vi "Distillation Column #2.vi"() -> ()   [LabVIEW 2017]
uses:
  Halt BioReact.vi
panel:
  in  "Cooling Water Setpoint":dbl caption="L/hr"
  in  "Main Power":bool
  out "Feed Scale":dbl caption="kg" format="%.4f"
  out "Cooling Water Flowrate":dbl caption="L/hr" format="%.1f"
  out "Reboiler Pressure":dbl caption="\"WC" format="%.1f"
  in  "stop":bool
  out "Data Point Count":i32
  in  "Specify Time between Data Points (sec)":dbl=1.0
  in  "Cancel Data Collection":bool
  in  "Specify number of data points":i16=1
  in  "Enable 3":bool
  out "Saving Data 3":bool
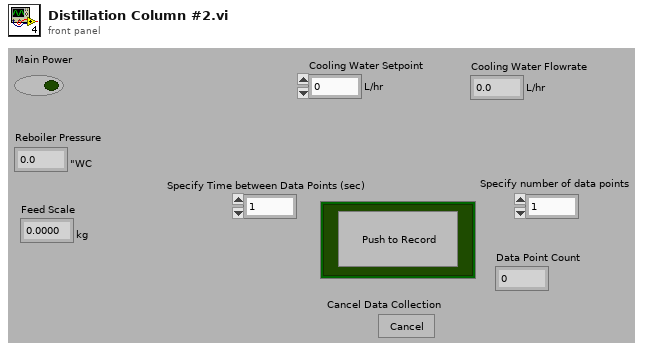
[diagram p1: front panel]
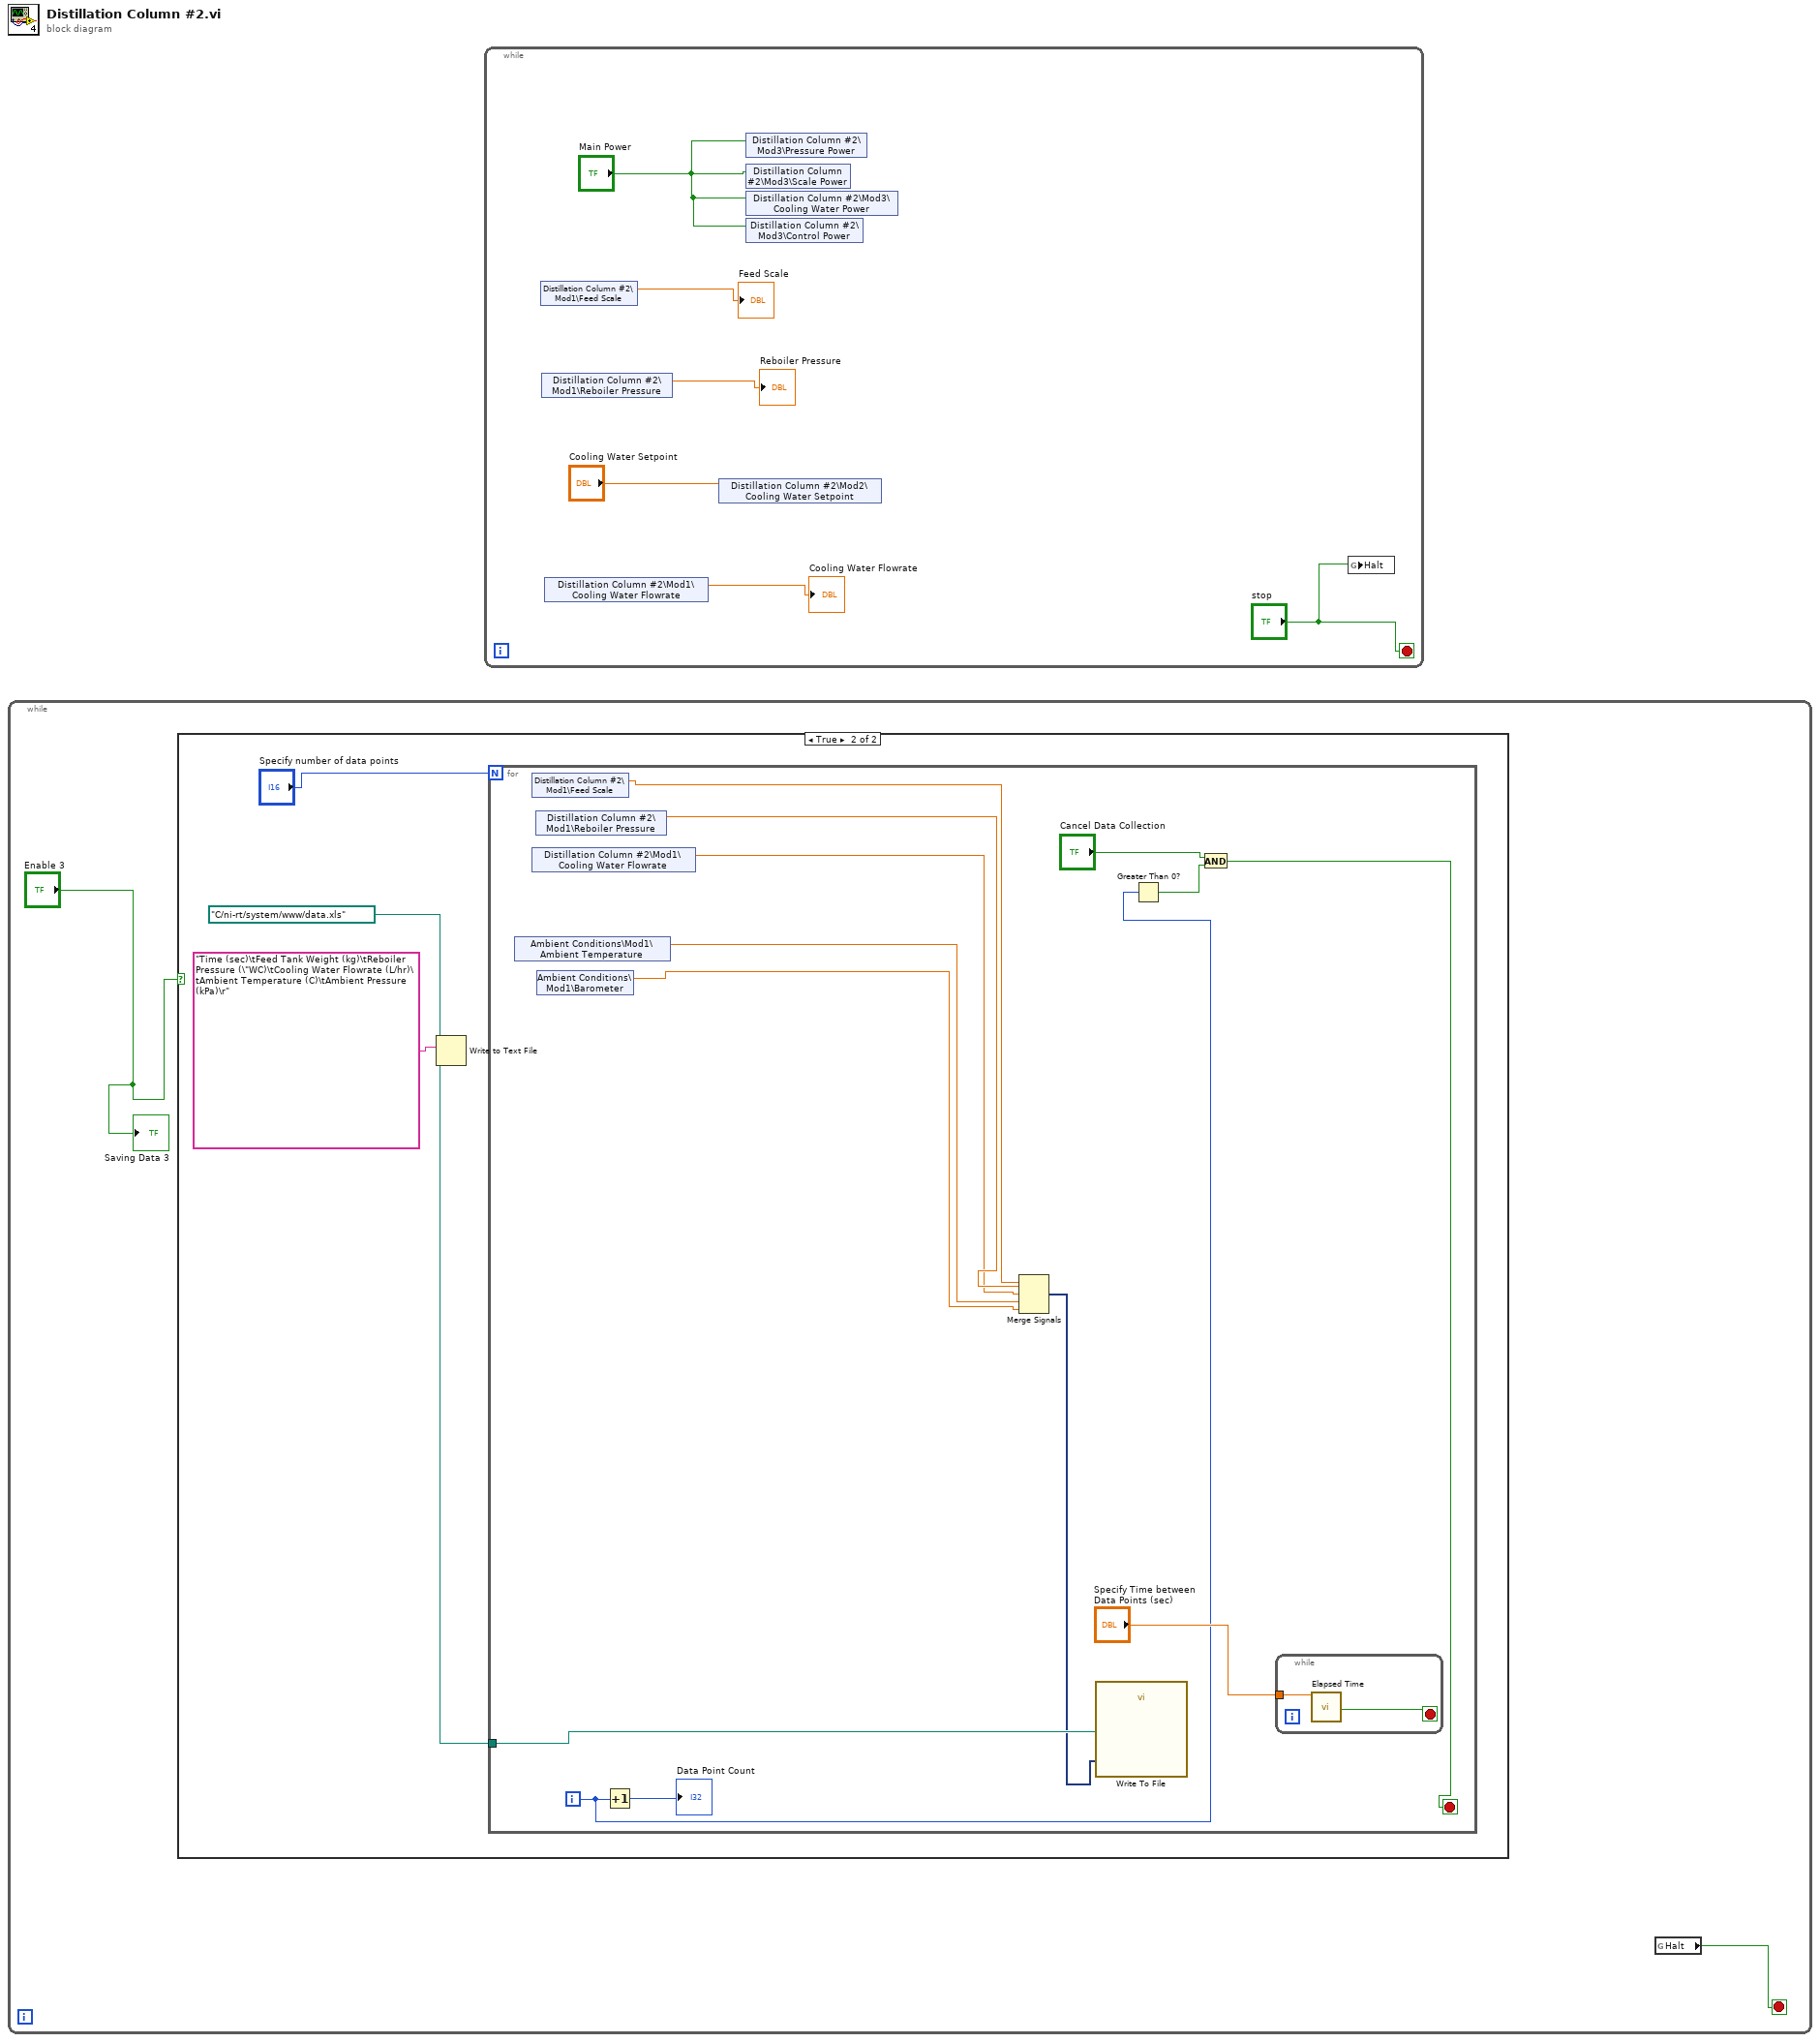
[diagram p0: block diagram]
diagram:
  n1 = while {
    stop <- w1 stop-if-true
    n2 = case shown="True" "Enable 3" {
      frame False {
      }
      frame True {
        w4 = path "C:/ni-rt/system/www/data.xls" ("Filename")
        n3 = Write to Text File(file (use dialog)=w4, text="Time (sec)\tFeed Tank Weight (kg)\tReboiler Pressure (\"WC)\tCooling Water Flowrate (L/hr)\tAmbient Temperature (C)\tAmbient Pressure (kPa)\r") -> ()  [unwired: 2 in, 3 out]
        n4 = for {
          N: "Specify number of data points" -> [_]
          tunnel: w4 -> [w18]
          i -> [w14]
          stop <- w11 stop-if-true
          n5 = shared-variable "Ambient Conditions\\Mod1\\Ambient Temperature"() -> (w10:dbl)  [unwired: 1 in, 1 out]
          n6 = shared-variable "Distillation Column #2\\Mod1\\Feed Scale"() -> (w8:dbl)  [unwired: 1 in, 1 out]
          n7 = shared-variable "Distillation Column #2\\Mod1\\Cooling Water Flowrate"() -> (w6:dbl)  [unwired: 1 in, 1 out]
          n8 = shared-variable "Distillation Column #2\\Mod1\\Reboiler Pressure"() -> (w7:dbl)  [unwired: 1 in, 1 out]
          n9 = shared-variable "Ambient Conditions\\Mod1\\Barometer"() -> (w9:dbl)  [unwired: 1 in, 1 out]
          n10 = Increment(x=w14) -> (x+1=→"Data Point Count":i32)
          n11 = Merge Signals(w8, w7, w6, w10, w9) -> (w16:dynamicdata)
          n12 = call "Write To File"("Signals"=w16, "Filename"=w18) -> ()  [unwired: 15 in, 3 out]
          n13 = Greater Than 0?(x=w14) -> (x > 0?=w12:bool)
          n14 = And(x="Cancel Data Collection", y=w12) -> (x .and. y?=w11:bool)
          n15 = while {
            tunnel: "Specify Time between Data Points (sec)" -> [w19]
            stop <- w20 stop-if-true
            n16 = call "Elapsed Time"("Time Target (s)"=w19) -> ("Time has Elapsed"=w20:bool)  [unwired: 11 in, 7 out]
          }
        }
      }
    }
    n17 = global read "Halt BioReact.vi" "Halt"() -> (w1:bool)
    "Saving Data 3" <- "Enable 3"
  }
  n18 = while {
    stop <- "stop" stop-if-true
    n19 = shared-variable "Distillation Column #2\\Mod1\\Feed Scale"() -> (→"Feed Scale":dbl)  [unwired: 1 in, 1 out]
    n20 = shared-variable "Distillation Column #2\\Mod1\\Reboiler Pressure"() -> (→"Reboiler Pressure":dbl)  [unwired: 1 in, 1 out]
    n21 = shared-variable "Distillation Column #2\\Mod1\\Cooling Water Flowrate"() -> (→"Cooling Water Flowrate":dbl)  [unwired: 1 in, 1 out]
    n22 = shared-variable "Distillation Column #2\\Mod2\\Cooling Water Setpoint"("Cooling Water Setpoint") -> ()  [unwired: 1 in, 1 out]
    n23 = shared-variable "Distillation Column #2\\Mod3\\Pressure Power"("Main Power") -> ()  [unwired: 1 in, 1 out]
    n24 = shared-variable "Distillation Column #2\\Mod3\\Scale Power"("Main Power") -> ()  [unwired: 1 in, 1 out]
    n25 = shared-variable "Distillation Column #2\\Mod3\\Cooling Water Power"("Main Power") -> ()  [unwired: 1 in, 1 out]
    n26 = shared-variable "Distillation Column #2\\Mod3\\Control Power"("Main Power") -> ()  [unwired: 1 in, 1 out]
    n27 = global write "Halt BioReact.vi" "Halt"("stop") -> ()
  }
